vi "Execute.vi"(8 "error in":errorcluster, 11 "Set cycle state STEP in":refnum<class "Reset cycle state STEP.lvclass">) -> (0 "error out":errorcluster, 1 "Next Step?":bool, 2 "MSG":string, 3 "Set cycle state STEP out":refnum<class "Reset cycle state STEP.lvclass">)   [LabVIEW 2014, in "Reset cycle state STEP.lvclass"]
uses:
  Reset cycle state STEP.lvclass
  <vilib>/ActorFramework/Message Enqueuer/Message Enqueuer.lvclass
  Controller/Messages/Toggle Filter Cycle/Toggle Filter Cycle MSG.lvclass
  Controller/Messages/Toggle Speaker Cycle/Toggle Speaker Cycle MSG.lvclass
  reusable/Sequence/STEPS/STEP.lvclass/STEP.ctl
  Controller/Messages/Toggle Filter Cycle/Toggle Filter Cycle MSG.lvclass/Toggle Filter Cycle MSG.ctl
  Controller/Messages/Toggle Speaker Cycle/Toggle Speaker Cycle MSG.lvclass/Toggle Speaker Cycle MSG.ctl
  <vilib>/ActorFramework/Message Enqueuer/Message Enqueuer.lvclass/Message Enqueuer.ctl
  reusable/Sequence/STEPS/Read Obj.vi
  Controller/Messages/Toggle Filter Cycle/Write Cycle_.vi
  Controller/Messages/Toggle Speaker Cycle/Write Cycle_.vi
  <vilib>/ActorFramework/Message Priority Queue/Priority Enqueue.vi
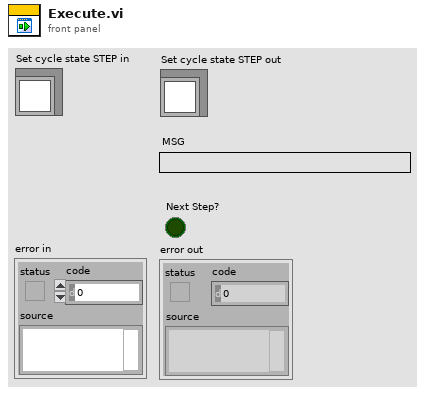
[diagram p1: front panel]
types:
  T1 = cluster{"Cycle":bool, "Period":i16, "Length":i16}
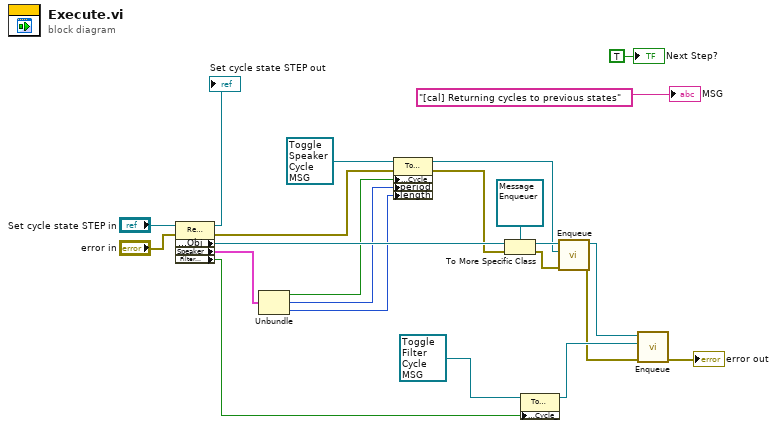
[diagram p0: block diagram]
diagram:
  n1 = property class="Reset cycle state STEP.lvclass"(reference="Set cycle state STEP in", error in="error in") -> (reference out=→"Set cycle state STEP out":refnum<class "Reset cycle state STEP.lvclass">, error out=w18:errorcluster, "Accessors:Obj"=w23:refnum<class>, "Speaker"=w4:T1, "Filter Cycle"=w5:bool)
  n2 = Unbundle(w4) -> ("Cycle"=w3:bool, "Period"=w2:i16, "Length"=w1:i16)
  n3 = property class="Toggle Speaker Cycle MSG"(reference=refnum<class "Toggle Speaker Cycle MSG.lvclass"> refnum ("Controller:Toggle Speaker Cycle MSG"), error in=w18, "Accessors:Cycle_"=w3, "period"=w2, "length"=w1) -> (reference out=w19:refnum<class "Toggle Speaker Cycle MSG.lvclass">, error out=w17:errorcluster)
  n4 = To More Specific Class(target class=refnum<class "Message Enqueuer.lvclass"> refnum ("Message Enqueuer in"), reference=w23, error in=w17) -> (specific class reference=w20:refnum<class "Message Enqueuer.lvclass">, error out=w21:errorcluster)
  n5 = property class="Toggle Filter Cycle"(reference=refnum<class "Toggle Filter Cycle MSG.lvclass"> refnum ("Controller:Toggle Filter Cycle MSG.lvclass"), "Accessors:Cycle_"=w5) -> (reference out=w9:refnum<class "Toggle Filter Cycle MSG.lvclass">)  [unwired: 1 in, 1 out]
  n6 = call <vilib>:"Enqueue.vi"("error in (no error)"=w21, "Message"=w19, "Message Enqueuer in"=w20) -> ("error out"=w8:errorcluster, "Message Enqueuer out"=w10:refnum<class "Message Enqueuer.lvclass">)  [unwired: 7 in]
  n7 = call <vilib>:"Enqueue.vi"("error in (no error)"=w8, "Message"=w9, "Message Enqueuer in"=w10) -> ("error out"=→"error out":errorcluster)  [unwired: 7 in, 1 out]
  "Next Step?" <- TRUE ("Next Step?")
  "MSG" <- "[cal] Returning cycles to previous states" ("format string")
